vi "KH TURCK ETHERNETIP RFID UserCommand Array.vi"(8 "BitArray":bool[](array[boolean]), 10 "UserCommand":T1, 11 "TagNr":enum16{"Tag 0", "Tag 1"}(ring)) -> (0 "index of element":i32, 3 "initialized array":bool[](array[boolean]))   [LabVIEW 2021]
uses:
  KH TURCK ETHERNETIP TDef Enum RFID User Command.ctl
  KH TURCK ETHERNETIP RFID Global.vi
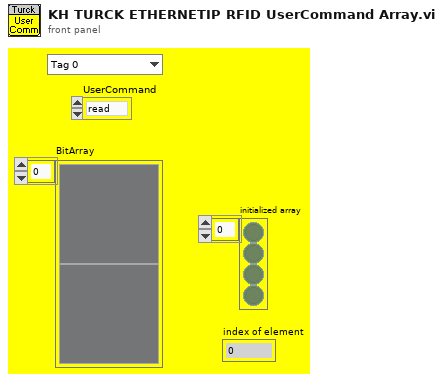
[diagram p1: front panel]
types:
  T1 = typedef "KH TURCK ETHERNETIP TDef Enum RFID User Command.ctl" = enum16{"read", "write", "idle", "inventory"}
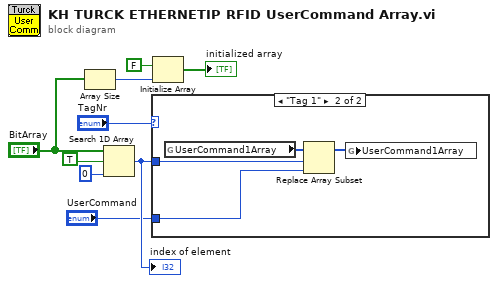
[diagram p0: block diagram]
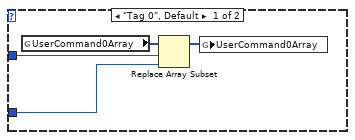
[diagram p2: hidden frame]
diagram:
  n1 = Array Size(array="BitArray") -> (size(s)=w3:i32)
  n2 = Search 1D Array(1D array="BitArray", element=TRUE, start index (0)=0) -> (index of element=w7:i32)
  "index of element" <- w7
  n3 = case shown="\"Tag 1\"" "TagNr" {
    tunnel: w7 -> [w12 w15]
    tunnel: "UserCommand" -> [w10 w14]
    frame "Tag 0", Default {
      n4 = global read "KH TURCK ETHERNETIP RFID Global.vi" "UserCommand0Array"() -> (w13:T1[])
      n5 = Replace Array Subset(array=w13, new element=w10, index=w12) -> (w11:T1[])
      n6 = global write "KH TURCK ETHERNETIP RFID Global.vi" "UserCommand0Array"(w11) -> ()
    }
    frame "Tag 1" {
      n7 = global read "KH TURCK ETHERNETIP RFID Global.vi" "UserCommand1Array"() -> (w17:T1[])
      n8 = Replace Array Subset(array=w17, new element=w14, index=w15) -> (w16:T1[])
      n9 = global write "KH TURCK ETHERNETIP RFID Global.vi" "UserCommand1Array"(w16) -> ()
    }
  }
  n10 = Initialize Array(FALSE ("element"), w3) -> (→"initialized array":bool[])
